vi "Read Data as Mono14 Image.vi"(8 "error in (no error)":errorcluster, 11 "Buffer in":refnum<class "Buffer.lvclass">) -> (0 "error out":errorcluster, 2 "Image":u16[][](array[numeric]), 3 "Buffer":refnum<class "Buffer.lvclass">)   [LabVIEW 2020, in "Buffer.lvclass"]
uses:
  Buffer.lvclass
  Buffer.lvclass/Buffer.ctl
  <vilib>/Utility/error.llb/Error Cluster From Error Code.vi
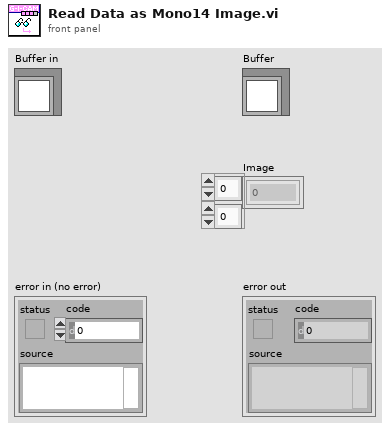
[diagram p1: front panel]
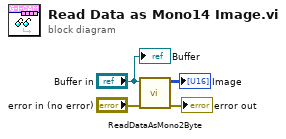
[diagram p0: block diagram]
diagram:
  n1 = call "ReadDataAsMono2Byte.vi"("error in (no error)"="error in (no error)", "Buffer in"="Buffer in") -> ("error out"=→"error out":errorcluster, "Image"=→"Image":u16[][])  [unwired: 8 in]
  "Buffer" <- "Buffer in"
